vi "PDash - Convert DQMH Event.vi"(6 "New Event Type":T1, 9 "New Broadcast Name":string, 10 "Event Info (Converted)":T2={"Event VI Path"=path "", "Argument Path"=path "", "Wait Argument Path"=path "", "Event Arg Owner"=-1, "Event Name"="", "Type"=enum."Request"}, 11 "Module Info":T4) -> (0 "error out":errorcluster)   [LabVIEW 2020]
doc: "_____\nCreated using DQMH Event Scripter 7.1.0.1447."
uses:
  <vilib>/Delacor/Delacor QMH/Libraries/_Scripting Support/Module Info--cluster.ctl
  <vilib>/Delacor/Delacor QMH/Libraries/_Scripting Support/Module Type--enum.ctl
  <vilib>/Delacor/Delacor QMH/Libraries/_Scripting Support/Event Info (Existing)--cluster.ctl
  Program Files (x86)/National Instruments/LabVIEW 2020/project/Delacor/DQMH/_DQMH Remove Event/Event Type (All Permutations)--enum.ctl
  <vilib>/Delacor/Delacor QMH/Libraries/_Scripting Support/Event Type (Convert)--enum.ctl
  PantherDashboard Scripting Hooks/Panther Dasboard Scripting Hooks.lvlib
  <vilib>/Delacor/Delacor QMH/Libraries/_Scripting Support/dqmh_lib_DQMH Scripting Support.lvlib
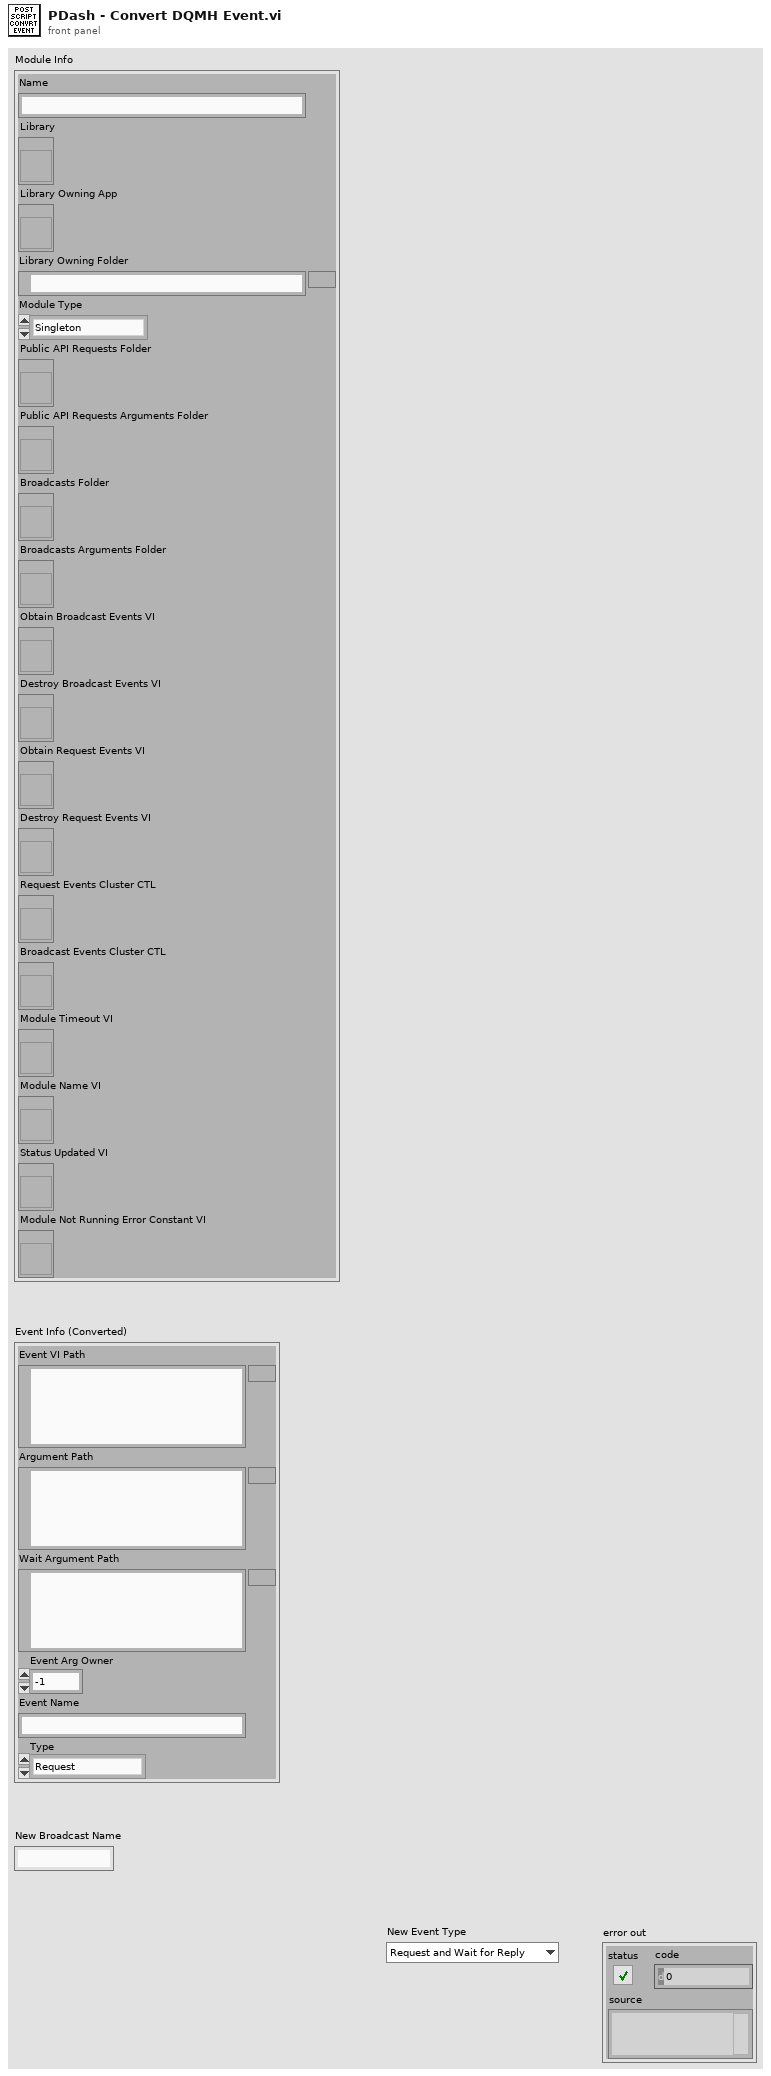
[diagram p1: front panel]
types:
  T1 = typedef "dqmh_lib_DQMH Scripting Support.lvlib/Event Type (Convert)--enum.ctl" = enum16{"Request and Wait for Reply", "Round Trip"}
  T2 = typedef "dqmh_lib_DQMH Scripting Support.lvlib/Event Info (Existing)--cluster.ctl" = cluster{"Event VI Path":path, "Argument Path":path, "Wait Argument Path":path, "Event Arg Owner":i32, "Event Name":string, "Type":T3}
  T3 = typedef "dqmh_lib_DQMH Scripting Support.lvlib/Event Type (All Permutations)--enum.ctl" = enum16{"Request", "Broadcast", "Both", "Request (no Wait)", "Request and Wait", "Request (Private)", "Request (Local Instance)"}
  T4 = typedef "dqmh_lib_DQMH Scripting Support.lvlib/Module Info--cluster.ctl" = cluster{"Name":string, "Library":refnum<vi>, "Library Owning App":refnum<vi>, "Library Owning Folder":path, "Module Type":T5, "Public API Requests Folder":refnum<vi>, "Public API Requests Arguments Folder":refnum<vi>, "Broadcasts Folder":refnum<vi>, "Broadcasts Arguments Folder":refnum<vi>, "Obtain Broadcast Events VI":refnum<vi>, "Destroy Broadcast Events VI":refnum<vi>, "Obtain Request Events VI":refnum<vi>, "Destroy Request Events VI":refnum<vi>, "Request Events Cluster CTL":refnum<vi>, "Broadcast Events Cluster CTL":refnum<vi>, "Module Timeout VI":refnum<vi>, "Module Name VI":refnum<vi>, "Status Updated VI":refnum<vi>, "Module Not Running Error Constant VI":refnum<vi>}
  T5 = typedef "dqmh_lib_DQMH Scripting Support.lvlib/Module Type--enum.ctl" = enum16{"Singleton", "Cloneable"}
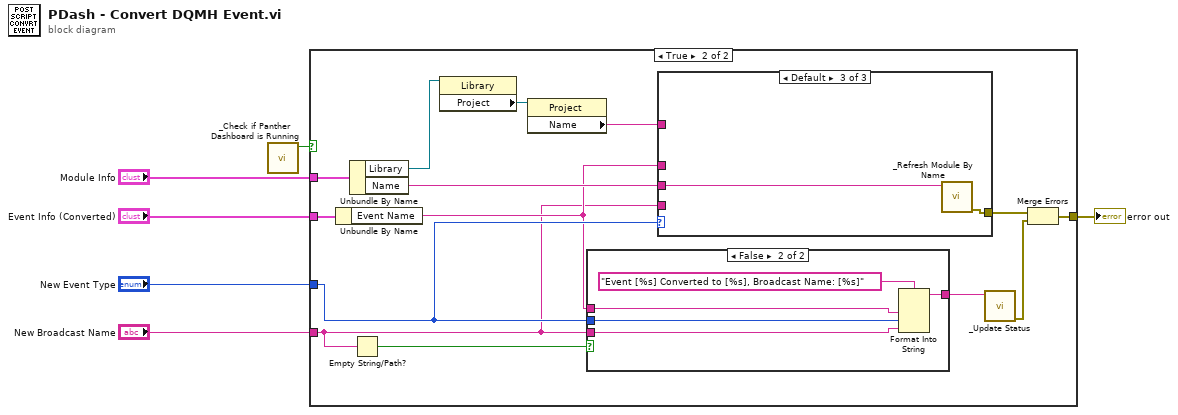
[diagram p0: block diagram]
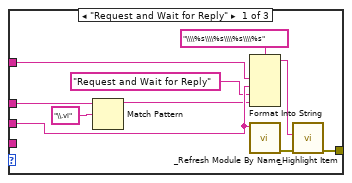
[diagram p3: hidden frame]
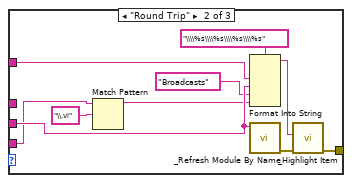
[diagram p4: hidden frame]
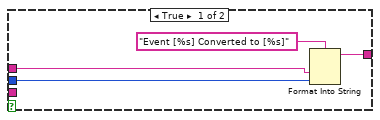
[diagram p5: hidden frame]
diagram:
  n1 = call "_Check if Panther Dashboard is Running.vi"() -> ("Panther Dashboard is Running?"=w2:bool)  [unwired: 10 in, 1 out]
  n2 = case shown="True" w2 {
    tunnel: [_ w19] -> w6
    tunnel: "Event Info (Converted)" -> [_ w10]
    tunnel: "New Event Type" -> [_ w9]
    tunnel: "New Broadcast Name" -> [_ w7]
    tunnel: "Module Info" -> [_ w11]
    frame False {
    }
    frame True {
      n3 = Unbundle By Name(w10) -> ("Event Name"=w8:string)
      n4 = Unbundle By Name(w11) -> ("Library"=w13:refnum<vi>, "Name"=w12:string)
      n5 = Empty String/Path?(string/path=w7) -> (empty?=w17:bool)
      n6 = property class="Library"(reference=w13) -> ("Project"=w15:refnum<vi>)  [unwired: 1 in, 2 out]
      n7 = property class="Project"(reference=w15) -> ("Name"=w14:string)  [unwired: 1 in, 2 out]
      n8 = case shown="False" w17 {
        tunnel: [w46 w51] -> w16
        tunnel: w8 -> [w45 w50]
        tunnel: w9 -> [w44 w49]
        tunnel: w7 -> [_ w47]
        frame True {
          n9 = Format Into String(format string="Event [%s] Converted to [%s]", w45, w44) -> (resulting string=w46:string)  [unwired: 2 in, 1 out]
        }
        frame False {
          n10 = Format Into String(format string="Event [%s] Converted to [%s], Broadcast Name: [%s]", w50, w49, w47) -> (resulting string=w51:string)  [unwired: 2 in, 1 out]
        }
      }
      n11 = case shown="Default" w9 {
        tunnel: [w29 w39 w42] -> w18
        tunnel: w14 -> [w28 w38 _]
        tunnel: w12 -> [w25 w35 w41]
        tunnel: w8 -> [w24 _ _]
        tunnel: w7 -> [_ w31 _]
        frame "Request and Wait for Reply" {
          n12 = Match Pattern(string=w24, regular expression="\\.vi") -> (before substring=w23:string)  [unwired: 1 in, 3 out]
          n13 = Format Into String(format string="\\\\%s\\\\%s\\\\%s\\\\%s", w28, w25, "Request and Wait for Reply", w23) -> (resulting string=w27:string)  [unwired: 2 in, 1 out]
          n14 = call "_Refresh Module By Name.vi"("Module Name"=w25) -> ("error out"=w30:errorcluster)  [unwired: 10 in]
          n15 = call "_Highlight Item.vi"("error in"=w30, "Item Tag"=w27) -> ("error out"=w29:errorcluster)  [unwired: 9 in]
        }
        frame "Round Trip" {
          n16 = Match Pattern(string=w31, regular expression="\\.vi") -> (before substring=w34:string)  [unwired: 1 in, 3 out]
          n17 = Format Into String(format string="\\\\%s\\\\%s\\\\%s\\\\%s", w38, w35, "Broadcasts", w34) -> (resulting string=w37:string)  [unwired: 2 in, 1 out]
          n18 = call "_Refresh Module By Name.vi"("Module Name"=w35) -> ("error out"=w40:errorcluster)  [unwired: 10 in]
          n19 = call "_Highlight Item.vi"("error in"=w40, "Item Tag"=w37) -> ("error out"=w39:errorcluster)  [unwired: 9 in]
        }
        frame Default {
          n20 = call "_Refresh Module By Name.vi"("Module Name"=w41) -> ("error out"=w42:errorcluster)  [unwired: 10 in]
        }
      }
      n21 = call "_Update Status.vi"("Status"=w16) -> ("error out"=w20:errorcluster)  [unwired: 10 in]
      n22 = Merge Errors(w18, w20) -> (w19:errorcluster)
    }
  }
  "error out" <- w6
